vi "RunAllTests.vi"() -> ()   [LabVIEW 2019]
doc: "JKI State Machine Objects (SMO) 1.0.0.5\nJKI - JKI\nCopyright (c) 2016, JKI"
uses:
  TestInheritance/TestNoSubpanels.lvclass
  C:/Program Files (x86)/National Instruments/LabVIEW 2019/vi.lib/JKI/JKI SMO/SMO/SMO.lvclass
  C:/Program Files (x86)/National Instruments/LabVIEW 2019/vi.lib/JKI/JKI SMO/SMO.UI/SMO.UI.lvclass
  TestDefaultDirectory/Maui.Test.DefaultDirectory.lvclass
  <vilib>/JKI/JKI SMO/SMO/SMO.lvclass/SMO.ctl
  <vilib>/JKI/JKI SMO/SMO.UI/SMO.UI.lvclass/SMO.UI.ctl
  <vilib>/JKI/JKI SMO/SMO/Typedefs/SMOState --Enum.ctl
  <vilib>/JKI/JKI SMO/SMO/Private/ReftoDVR--SMO.vi
  <vilib>/JKI/JKI SMO/SMO.UI/SMO.UI.ReftoDVR.vi
  <vilib>/JKI/JKI SMO/SMO/SMO.lvclass
  <vilib>/JKI/JKI SMO/SMO.UI/SMO.UI.lvclass
panel:
  out "error out":errorcluster
  in  "Stop":bool
  # "Run All Tests"
  # "For instructions on how to use the JKI State Machine Objects, examples and video tutorials, visit:\nhttp://jki.net/state-machine-objects/\n\nJKI State Machine Objects™\nhttp://jki.net/state-machine-objects/\nCopyright (C) 2005-2015, JKI <info@jki.net>\nALL RIGHTS RESERVED"
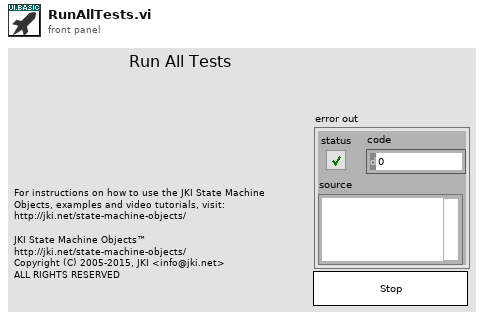
[diagram p1: front panel]
types:
  T1 = typedef "SMO.lvclass/Public Events.ctl" = cluster{"Error":refnum<user-event>, "State":refnum<user-event>, "Reserve State":refnum<user-event>}
  T2 = typedef "SMO.UI.lvclass/PublicEvents--Cluster.ctl" = cluster{"UI Hidden":refnum<user-event>, "UI State":refnum<user-event>}
  T3 = typedef "SMO.lvclass/SMOState --Enum.ctl" = enum16{"unknown", "Created", "Started", "Stopped"}
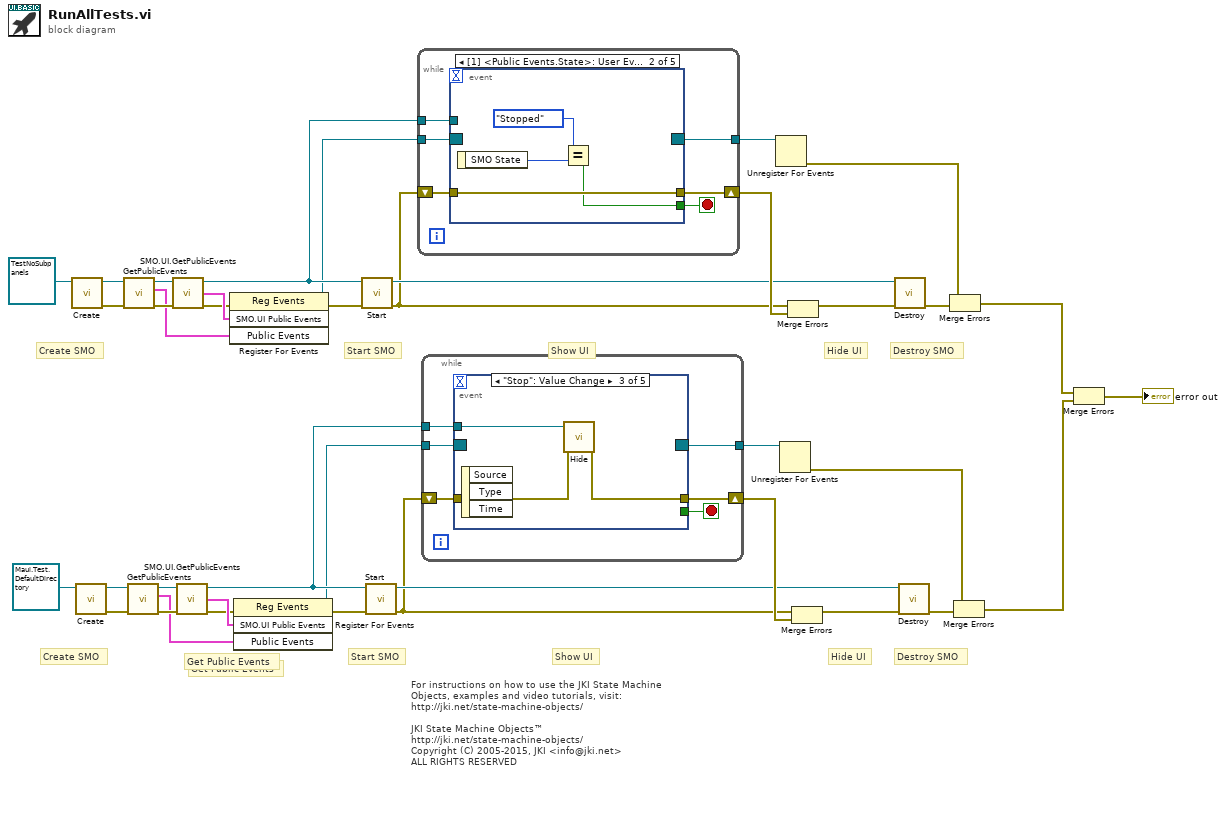
[diagram p0: block diagram]
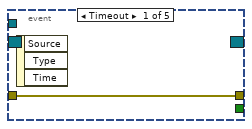
[diagram p2: hidden frame]
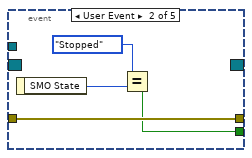
[diagram p3: hidden frame]
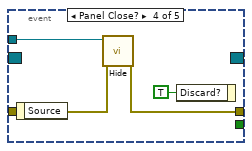
[diagram p4: hidden frame]
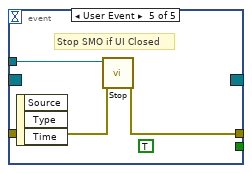
[diagram p5: hidden frame]
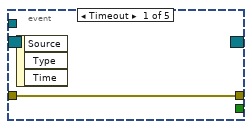
[diagram p6: hidden frame]
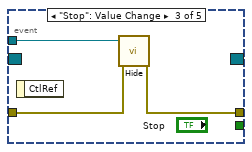
[diagram p7: hidden frame]
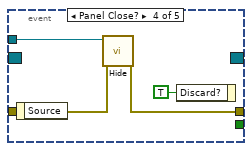
[diagram p8: hidden frame]
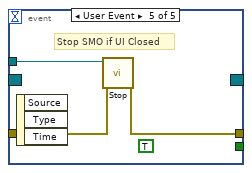
[diagram p9: hidden frame]
diagram:
  # "Hide UI"
  # "Show UI"
  # "Get Public Events"
  # "Start SMO"
  # "Destroy SMO"
  # "Create SMO"
  # "Hide UI"
  # "Show UI"
  # "For instructions on how to use the JKI State Machine Objects, examples and video tutorials, visit:\nhttp://jki.net/state-machine-objects/\n\nJKI State Machine Objects™\nhttp://jki.net/state-machine-objects/\nCopyright (C) 2005-2015, JKI <info@jki.net>\nALL RIGHTS RESERVED"
  # "Get Public Events"
  # "Start SMO"
  # "Destroy SMO"
  # "Create SMO"
  n1 = call <vilib>:"Create.vi"("SMO"=refnum<class "TestNoSubpanels.lvclass"> refnum ("SMO.Template.lvclass")) -> ("error out"=w26:errorcluster, "SMO out"=w25:refnum<class "TestNoSubpanels.lvclass">)  [unwired: 8 in, 1 out]
  n2 = call <vilib>:"Create.vi"("SMO"=refnum<class "Maui.Test.DefaultDirectory.lvclass"> refnum ("SMO.Template.lvclass")) -> ("error out"=w8:errorcluster, "SMO out"=w7:refnum<class "Maui.Test.DefaultDirectory.lvclass">)  [unwired: 8 in, 1 out]
  n3 = call <vilib>:"GetPublicEvents.vi"("error in (no error)"=w26, "SMO"=w25) -> ("error out"=w23:errorcluster, "Public Events"=w22:T1, "SMO out"=w24:refnum<class "TestNoSubpanels.lvclass">)  [unwired: 7 in]
  n4 = call <vilib>:"GetPublicEvents.vi"("error in (no error)"=w8, "SMO"=w7) -> ("error out"=w5:errorcluster, "Public Events"=w4:T1, "SMO out"=w6:refnum<class "Maui.Test.DefaultDirectory.lvclass">)  [unwired: 7 in]
  n5 = call <vilib>:"SMO.UI.GetPublicEvents.vi"("error in (no error)"=w23, "SMO.UI"=w24) -> ("error out"=w29:errorcluster, "SMO.UI Public Events"=w30:T2, "SMO.UI out"=w31:refnum<class "TestNoSubpanels.lvclass">)  [unwired: 7 in]
  n6 = call <vilib>:"SMO.UI.GetPublicEvents.vi"("error in (no error)"=w5, "SMO.UI"=w6) -> ("error out"=w11:errorcluster, "SMO.UI Public Events"=w12:T2, "SMO.UI out"=w13:refnum<class "Maui.Test.DefaultDirectory.lvclass">)  [unwired: 7 in]
  n7 = register-events(error in=w29, w30, w22) -> (reference out=w27:refnum<event-registration>, error out=w28:errorcluster)  [unwired: 1 in]
  n8 = register-events(error in=w11, w12, w4) -> (reference out=w9:refnum<event-registration>, error out=w10:errorcluster)  [unwired: 1 in]
  n9 = call <vilib>:"Start.vi"("error in (no error)"=w28, "SMO"=w31) -> ("error out"=w33:errorcluster, "SMO out"=w34:refnum<class "TestNoSubpanels.lvclass">)  [unwired: 8 in]
  n10 = call <vilib>:"Start.vi"("error in (no error)"=w10, "SMO"=w13) -> ("error out"=w15:errorcluster, "SMO out"=w16:refnum<class "Maui.Test.DefaultDirectory.lvclass">)  [unwired: 8 in]
  n11 = while {
    shift-right: [w44] -> w38
    shift-left: w33 -> [w43]
    tunnel: w27 -> [w42]
    tunnel: [w41] -> w39
    tunnel: w31 -> [w40]
    stop <- w45 stop-if-true
    n12 = event shown="[1] <Public Events.State>: User Event" {
      selector: w42 -> [_ _ _ _ _]
      dyn-events: [_ _ _ _ _] -> w41
      timeout: _ -> [_ _ _ _ _]
      tunnel: [_ w47 _ _ _] -> w45
      tunnel: w40 -> [_ _ w53 w56 w60]
      tunnel: [w46 w50 w51 w54 w59] -> w44
      tunnel: w43 -> [w46 w50 w52 w55 w58]
      event Timeout {
        n13 = event-data() -> ()  [unwired: 1 in, 3 out]
      }
      event User Event {
        n14 = event-data() -> ("SMO State"=w49:T3)  [unwired: 1 in]
        n15 = Equal?(x=SMOState_--Enum."Stopped", y=w49) -> (x = y?=w47:bool)
      }
      event "Stop": Value Change {
        n16 = event-data() -> ()  [unwired: 1 in, 1 out]
        n17 = call <vilib>:"Hide.vi"("error in (no error)"=w52, "SMO.UI"=w53) -> ("error out"=w51:errorcluster)  [unwired: 8 in, 1 out]
      }
      event Panel Close? {
        n18 = event-data() -> ()  [unwired: 1 in, 1 out]
        n19 = call <vilib>:"Hide.vi"("error in (no error)"=w55, "SMO.UI"=w56) -> ("error out"=w54:errorcluster)  [unwired: 8 in, 1 out]
        n20 = event-data("Discard?"=TRUE ("OK")) -> ()  [unwired: 1 in, 1 out]
      }
      event User Event {
        (unwired) TRUE ("OK")
        # "Stop SMO if UI Closed"
        n21 = event-data() -> ()  [unwired: 1 in, 3 out]
        n22 = call <vilib>:"Stop.vi"("error in (no error)"=w58, "SMO"=w60) -> ("error out"=w59:errorcluster)  [unwired: 8 in, 1 out]
      }
    }
  }
  n23 = while {
    shift-right: [w65] -> w20
    shift-left: w15 -> [w64]
    tunnel: w9 -> [w63]
    tunnel: [w62] -> w21
    tunnel: w13 -> [w61]
    stop <- w66 stop-if-true
    n24 = event shown="[2] \"Stop\": Value Change" {
      selector: w63 -> [_ _ _ _ _]
      dyn-events: [_ _ _ _ _] -> w62
      timeout: _ -> [_ _ _ _ _]
      tunnel: [_ w68 _ _ _] -> w66
      tunnel: w61 -> [_ _ w74 w77 w81]
      tunnel: [w67 w71 w72 w75 w80] -> w65
      tunnel: w64 -> [w67 w71 w73 w76 w79]
      event Timeout {
        n25 = event-data() -> ()  [unwired: 1 in, 3 out]
      }
      event User Event {
        n26 = event-data() -> ("SMO State"=w70:T3)  [unwired: 1 in]
        n27 = Equal?(x=SMOState_--Enum."Stopped", y=w70) -> (x = y?=w68:bool)
      }
      event "Stop": Value Change {
        n28 = event-data() -> ()  [unwired: 1 in, 3 out]
        n29 = call <vilib>:"Hide.vi"("error in (no error)"=w73, "SMO.UI"=w74) -> ("error out"=w72:errorcluster)  [unwired: 8 in, 1 out]
      }
      event Panel Close? {
        n30 = event-data() -> ()  [unwired: 1 in, 1 out]
        n31 = call <vilib>:"Hide.vi"("error in (no error)"=w76, "SMO.UI"=w77) -> ("error out"=w75:errorcluster)  [unwired: 8 in, 1 out]
        n32 = event-data("Discard?"=TRUE ("OK")) -> ()  [unwired: 1 in, 1 out]
      }
      event User Event {
        (unwired) TRUE ("OK")
        # "Stop SMO if UI Closed"
        n33 = event-data() -> ()  [unwired: 1 in, 3 out]
        n34 = call <vilib>:"Stop.vi"("error in (no error)"=w79, "SMO"=w81) -> ("error out"=w80:errorcluster)  [unwired: 8 in, 1 out]
      }
    }
  }
  n35 = Unregister For Events(event registration refnum=w39) -> (error out=w37:errorcluster)  [unwired: 1 in]
  n36 = Unregister For Events(event registration refnum=w21) -> (error out=w19:errorcluster)  [unwired: 1 in]
  n37 = Merge Errors(w33, w38) -> (w32:errorcluster)
  n38 = Merge Errors(w15, w20) -> (w14:errorcluster)
  n39 = call <vilib>:"Destroy.vi"("error in (no error)"=w32, "SMO"=w34) -> ("error out"=w36:errorcluster)  [unwired: 9 in]
  n40 = call <vilib>:"Destroy.vi"("error in (no error)"=w14, "SMO"=w16) -> ("error out"=w18:errorcluster)  [unwired: 9 in]
  n41 = Merge Errors(w37, w36) -> (w3:errorcluster)
  n42 = Merge Errors(w19, w18) -> (w2:errorcluster)
  n43 = Merge Errors(w3, w2) -> (→"error out":errorcluster)
